vi "Gyro.vi"(10 "GyroDevRef in":T1 {"Sample Rate" min=0.25 max=100.0 step=0.25}, 11 "Gyro Reset Angle":bool) -> (2 "Angle":dbl, 3 "GyroDevRef out":T1 {"Sample Rate" min=0.25 max=100.0 step=0.25})   [LabVIEW 2016]
uses:
  <vilib>/Rock Robotics/WPI/Gyro/WPI_GyroDevRef.ctl
  <vilib>/Rock Robotics/SystemInterfaces/AI/FPGA_AIChannel.ctl
  <vilib>/Rock Robotics/SystemInterfaces/spilib/spi_bus.ctl
  <vilib>/Rock Robotics/Network Tables/NT Write Number.vi
  Robot Global Data.vi
panel:
  # "Analog"
  # "XRS"
  # "Analog"
  # "XRS"
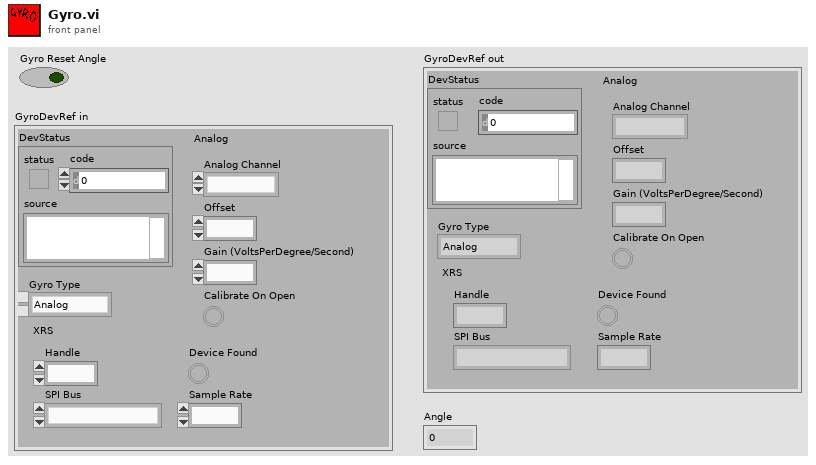
[diagram p1: front panel]
types:
  T1 = typedef "WPI_GyroDevRef.ctl" = cluster{"DevStatus":errorcluster, "Analog Channel":T2, "Offset":dbl, "Gain (VoltsPerDegree/Second)":dbl, "Gyro Type":enum16{"Analog", "XRS450"}, "Handle":i32, "SPI Bus":T3, "Device Found":bool, "Sample Rate":dbl, "Calibrate On Open":bool}
  T2 = typedef "FPGA_AIChannel.ctl" = enum8{"AI 0", "AI 1", "AI 2", "AI 3", "AI MXP 0", "AI MXP 1", "AI MXP 2", "AI MXP 3", "Invalid"}
  T3 = typedef "spi_bus.ctl" = enum16{"SPI On-Board, CS0", "SPI On-Board, CS1", "SPI On-Board, CS2", "SPI On-Board, CS3", "SPI MXP", "Invalid"}
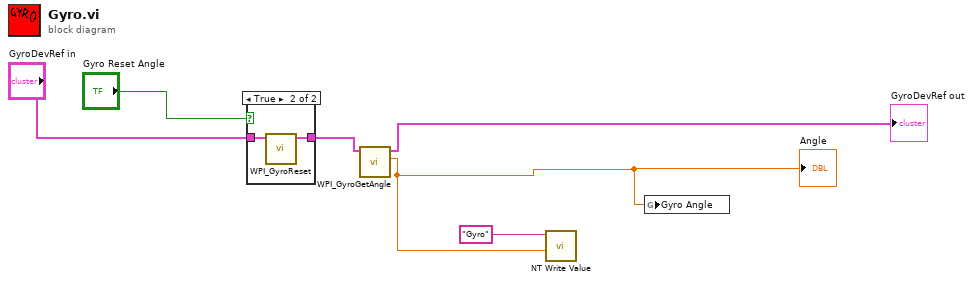
[diagram p0: block diagram]
diagram:
  n1 = case shown="True" "Gyro Reset Angle" {
    tunnel: "GyroDevRef in" -> [w7 w9]
    tunnel: [w7 w8] -> w4
    frame False {
    }
    frame True {
      n2 = call <vilib>:"WPI_GyroReset.vi"("GyroDevRef"=w9) -> ("GyroDevRef"=w8:T1)  [unwired: 9 in, 1 out]
    }
  }
  n3 = call <vilib>:"WPI_GyroGetAngle.vi"("GyroDevRef"=w4) -> ("Angle"=w1:dbl, "GyroDevRef"=→"GyroDevRef out":T1)  [unwired: 6 in, 3 out]
  "Angle" <- w1
  n4 = call-poly <vilib>:"NT Write Value.vi"("Numeric"=w1, "Name"="Gyro") -> ()  [unwired: 9 in, 1 out]
  n5 = global write "Robot Global Data.vi" "Gyro Angle"(w1) -> ()
